vi "Clear Plugin.vi"(8 "error in (no error)":errorcluster, 10 "Plugin":string, 11 "Execution UI in":refnum<class "Execution UI.lvclass">) -> (0 "error out":errorcluster, 3 "Execution UI out":refnum<class "Execution UI.lvclass">)   [LabVIEW 2020, in "Execution UI.lvclass"]
uses:
  Execution UI.lvclass
  Execution UI.lvclass/Execution UI.ctl
  Framework/Plugin/Plugin.lvclass
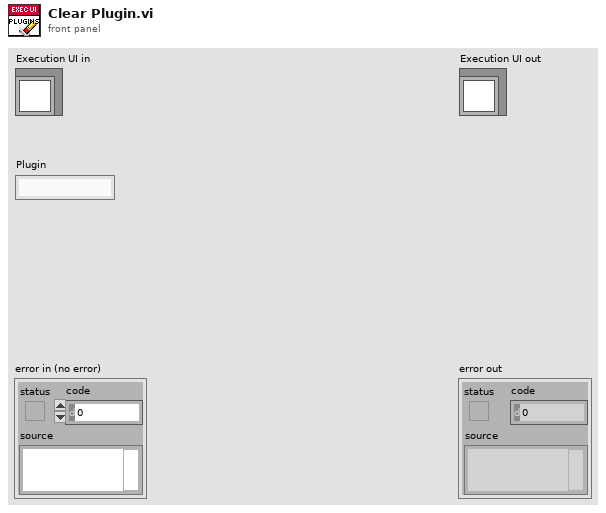
[diagram p1: front panel]
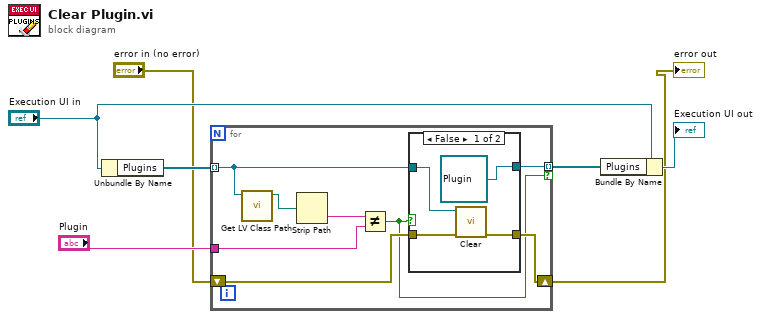
[diagram p0: block diagram]
diagram:
  n1 = Unbundle By Name("Execution UI in") -> ("Plugins"=w5:refnum<class "Plugin.lvclass">[])
  n2 = for {
    tunnel: w5 -> [w12] mode=indexing
    tunnel: "Plugin" -> [w13]
    shift-right: [w10] -> w2
    shift-left: "error in (no error)" -> [w11]
    tunnel: [w9] -> w1 mode=indexing if=w8
    n3 = call <vilib>:"Get LV Class Path.vi"("object"=w12) -> ("class path"=w15:path)  [unwired: 9 in, 1 out]
    n4 = Strip Path(path=w15) -> (name=w14:string)  [unwired: 1 out]
    n5 = Not Equal?(x=w14, y=w13) -> (x != y?=w8:bool)
    n6 = case shown="False" w8 {
      tunnel: w12 -> [w19 w20]
      tunnel: w11 -> [w18 w21]
      tunnel: [w17 w21] -> w10
      tunnel: [refnum<class "Plugin.lvclass"> refnum ("Plugin.lvclass") w20] -> w9
      frame False {
        n7 = call-dynamic "Clear.vi"("error in (no error)"=w18, "Plugin in"=w19) -> ("error out"=w17:errorcluster)  [unwired: 9 in]
      }
      frame True {
      }
    }
  }
  "error out" <- w2
  n8 = Bundle By Name(cluster="Execution UI in", "Plugins"=w1) -> (→"Execution UI out":refnum<class "Execution UI.lvclass">)
